vi "Dashboard Main.vi"() -> ()   [LabVIEW 2023]
uses:
  <vilib>/Rock Robotics/Network Tables/NT Read Numeric Array.vi
  <vilib>/Rock Robotics/Network Tables/NT Write Boolean.vi
  <vilib>/Rock Robotics/Network Tables/NT Write Number.vi
panel:
  out "Camera Perf":string
  in  "Camera Settings":T1={"Frame Rate"=30, "Compression"=30, "Size"=1, "DB Camera Config"=FALSE} {"Frame Rate" scale=1.0..30.0; "Compression" scale=100.0..-1.0; "Size" items=["640x480", "320x240", "160x120"]}
  in  "TCP":refnum<k5>
  out "Robot IP":string
  in  "Dashboard Tab":enum32{"Kilroy", "Variables", "Drive", "Basic"}(tab)
  in  "Auto Command Options":string(combo)
  in  "Demo Mode Enabled":bool
  in  "Auto Delay (seconds)":dbl(knob) min=0.0 max=5.0 scale=0.0..5.0 scale format="%#.2g"
  in  "Auto Selection":string(combo)
  in  "Auto Enabled":bool
  out "Tree":string(tree)
  in  "Select Auto":string(combo)="Select Autonomous ..."
  out "NT Connection":bool
  out "MotorChart R":cluster{"Numeric":dbl, "Numeric":dbl}(graph)
  out "MotorChart L":cluster{"Numeric":dbl, "Numeric":dbl}(graph)
  out "MotorSliders R":cluster{"MotorSlide1":dbl, "MotorSlide2":dbl} {"MotorSlide2" scale=-1.0..1.0 scale format="%#_2e"; "MotorSlide1" scale=-1.0..1.0 scale format="%#_2e"}
  out "MotorSliders L":cluster{"MotorSlide1":dbl, "MotorSlide2":dbl} {"MotorSlide2" scale=-1.0..1.0 scale format="%#_2e"; "MotorSlide1" scale=-1.0..1.0 scale format="%#_2e"}
  out "JS1 Z":dbl(slide) scale=-1.0..1.0 scale format="%#_2e"
  out "JS1 Graph":cluster{"X":dbl, "Y":dbl}[](graph)
  out "JS1 Buttons":T2
  out "JS2 Z":dbl(slide) scale=-1.0..1.0 scale format="%#_2e"
  out "JS2 Graph":cluster{"X":dbl, "Y":dbl}[](graph)
  out "JS2 Buttons":T2
  out "Mode":T3(ring)=enum."Auto Disabled"
  in  "DB/String 9":string
  in  "DB/String 8":string
  in  "DB/String 7":string
  in  "DB/String 6":string
  in  "DB/String 5":string
  in  "DB/String 4":string
  in  "DB/String 3":string
  in  "DB/String 2":string
  in  "DB/String 1":string
  in  "DB/String 0":string
  in  "DB/Slider 0":dbl(slide) scale=0.0..5.0
  in  "DB/Slider 1":dbl(slide) scale=0.0..5.0
  in  "DB/Slider 2":dbl(slide) scale=0.0..5.0
  in  "DB/Slider 3":dbl(slide) scale=0.0..5.0
  out "DB/LED 3":bool
  out "DB/LED 2":bool
  out "DB/LED 1":bool
  out "DB/LED 0":bool
  in  "DB/Button 3":bool
  in  "DB/Button 2":bool
  in  "DB/Button 1":bool
  in  "DB/Button 0":bool
  out "Camera Image":T4(plugin-control)
  out "Background":bool
  in  "Camera Name":string(combo)="No Camera Selection"
  # "HW"
  # "Joysticks"
  # "Drive Motors"
  # "Front"
  # "Right"
  # "Left"
  # "Back"
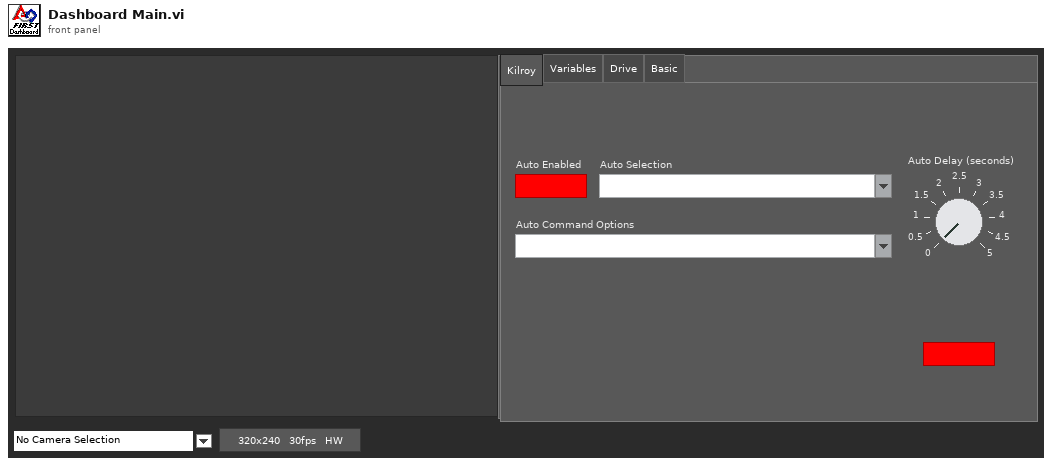
[diagram p1: front panel]
types:
  T1 = cluster{"Frame Rate":i32, "Compression":i32, "Size":u16, "DB Camera Config":bool}
  T2 = cluster{bool, bool, bool, bool, bool, bool, bool, bool, bool, bool, bool, bool}
  T3 = enum8{"Tele-Op Disabled", "Tele-Op Enabled", "Auto Disabled", "Auto Enabled", "Test Disabled", "Test Enabled", "Disconnected", "No Code", "E-Stop"}
  T4 = typedef "IMAQ Image.ctl" = refnum<image>
  T5 = cluster{"Save Path":path, "Interval (s)":dbl, "Keep":i32}
  T6 = typedef "Image Type" = u32
  T7 = cluster{"Camera Image":refnum<vi>, "Dashboard Tab":refnum<vi>, "Background":refnum<vi>, "Tree":refnum<vi>, "Camera Settings":refnum<vi>, "Camera Name":refnum<vi>, "Camera Perf":refnum<vi>}
  T8 = cluster{"Shift":bool, "Ctrl":bool, "Alt":bool, "Cmd":bool, "Opt":bool}
  T9 = cluster{"Error Strings":string, "Disable Counts":cluster{u16, u16}, "Rail Faults":cluster{u16, u16, u16}, "Robot IP":string, "DB Mode":u8, "Event Info":cluster{"Name":string, "Type":u8, "Number":u16, "Replay":u8}}
  T10 = cluster{"Storage":cluster{"Disk Free":u64, "RAM Block":u32, "RAM free":u32}, "CPU Utilization":cluster{"CPU % ISR":sgl, "CPU % Time Crit":sgl, "CPU % Timed Str":sgl, "CPU % High":sgl, "CPU % Above":sgl, "CPU % Normal":sgl, "CPU % Low":sgl}, "CAN":cluster{"% Bus Utilization":sgl, "Bus Off Cnt":u32, "TX_FIFO Full Cnt":u32, "Receive Error Cnt":u8, "Transmit Error Cnt":u8}, "HID":cluster{"HID Outputs":u32, "Rumble Low":u16, "Rumble High":u16}[]}
  T11 = cluster{"Status bits":cluster{"Test Mode":bool, "Autonomous":bool, "Enabled":bool, "Code Start":bool, "Brownout":bool, "Reserved 2":bool, "Reserved 3":bool, "E-Stop":bool}, "Code Trace":cluster{"Disabled":bool, "TeleOp":bool, "Auto":bool, "Test":bool}, "Controller Type":enum16{"unknown", "cRIO", "roboRio"}, "Code?":enum16{"unknown", "noCode", "code"}, "Battery V":dbl}
  T12 = cluster{"Control Bits":cluster{"TestMode":bool, "Autonomous":bool, "Enabled":bool, "FMS Present":bool, bool, bool, bool, "E-Stop":bool}, "Team Station ":u8, "Countdown":sgl, "Joystick Values":cluster{"Axes":dbl[], "Buttons":bool[], "POVs":i16[]}[]}
  T13 = cluster{"Axes":dbl[], "Buttons":bool[], "POVs":i16[]}[]
  T14 = cluster{"Axes":dbl[], "Buttons":bool[], "POVs":i16[]}
  T15 = cluster{"Buttons[0]":bool, "Buttons[1]":bool, "Buttons[2]":bool, "Buttons[3]":bool, "Buttons[4]":bool, "Buttons[5]":bool, "Buttons[6]":bool, "Buttons[7]":bool, "Buttons[8]":bool, "Buttons[9]":bool, "Buttons[10]":bool, "Buttons[11]":bool}
  T16 = cluster{"Camera Name":string, "Camera File Name":string, "Saved DB Images Info":cluster{"Save Path":path, "Interval (s)":dbl, "Keep":i32}}
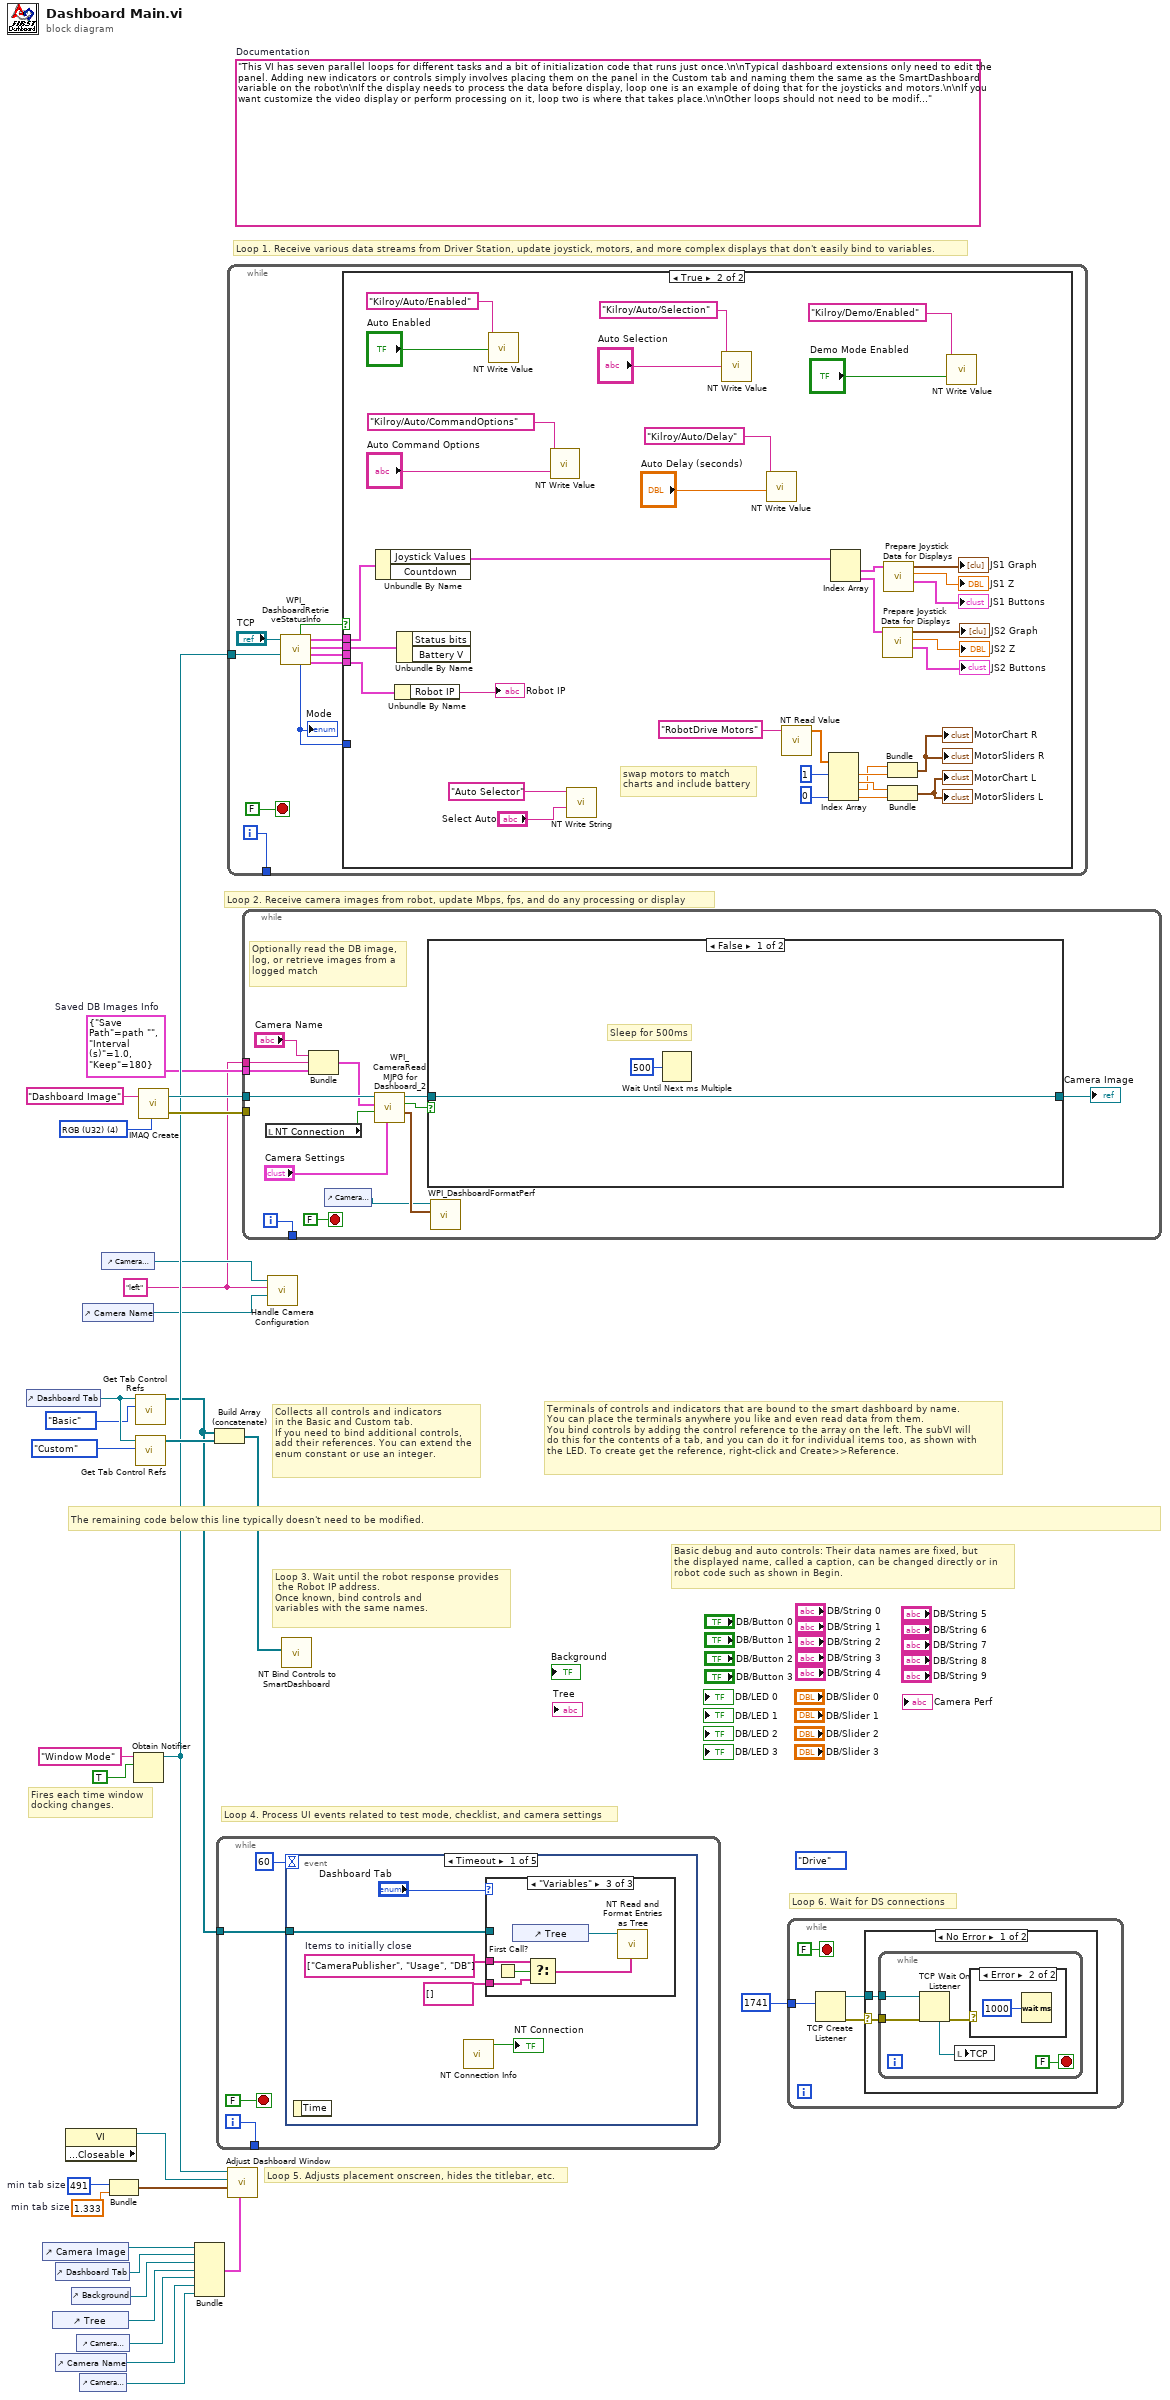
[diagram p0: block diagram]
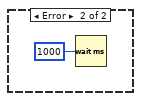
[diagram p3: hidden frame]
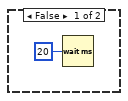
[diagram p4: hidden frame]
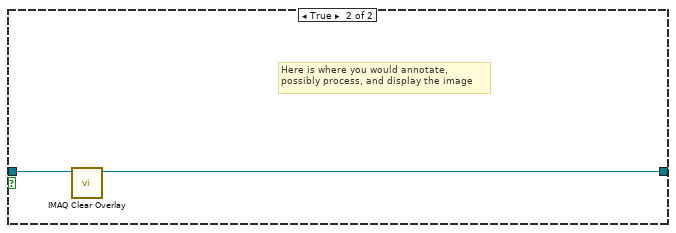
[diagram p5: hidden frame]
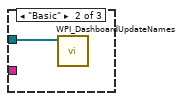
[diagram p7: hidden frame]
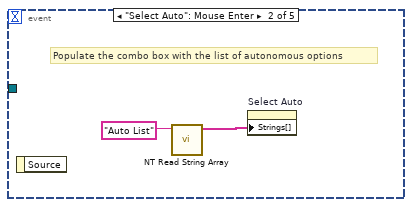
[diagram p8: hidden frame]
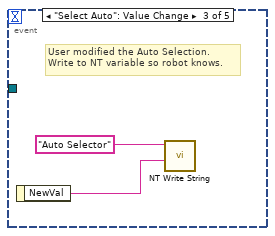
[diagram p9: hidden frame]
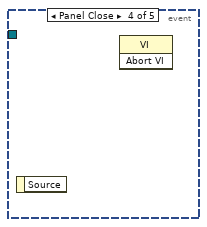
[diagram p10: hidden frame]
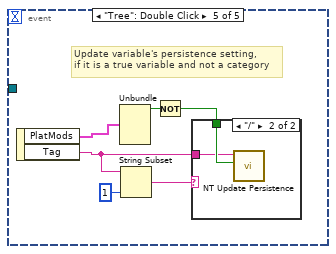
[diagram p11: hidden frame]
diagram:
  w2 = "left" ("Camera File Name")
  w3 = T5 {"Save Path"=path "", "Interval (s)"=1.0, "Keep"=180}  # Saved DB Images Info
  (unwired) enum32{"Drive", "Basic", "Custom", "Variables"}."Drive" ("Dashboard Tab")
  w18 = 491  # min tab size
  w17 = 1.333  # min tab size
  (unwired) "This VI has seven parallel loops for different tasks and a bit of initialization code that runs just once.\n\nTypical dashboard extensions only need to edit the panel. Adding new indicators or controls simply involves placing them on the panel in the Custom tab and naming them the same as the SmartDashboard variable on the robot\n\nIf the display needs to process the data before display, loop one is an example of doing that for the joysticks and motors.\n\nIf you want customize the video display or perform processing on it, loop two is where that takes place.\n\nOther loops should not need to be modified. They are pretty standard, and document the task they perform."  # Documentation
  w30 = T6 4 items=["Grayscale (U8)", "Grayscale (I16)", "Grayscale (SGL)", "Complex (CSG)", "RGB (U32)", "HSL (U32)", "RGB (U64)"] ("Image Type")
  # "Loop 6. Wait for DS connections"
  # "Basic debug and auto controls: Their data names are fixed, but\nthe displayed name, called a caption, can be changed directly or in\nrobot code such as shown in Begin."
  # "Fires each time window\ndocking changes."
  # "Collects all controls and indicators\nin the Basic and Custom tab.\nIf you need to bind additional controls,\nadd their references. You can extend the\nenum constant or use an integer."
  # "The remaining code below this line typically doesn't need to be modified."
  # "Loop 4. Process UI events related to test mode, checklist, and camera settings"
  # "Terminals of controls and indicators that are bound to the smart dashboard by name.\nYou can place the terminals anywhere you like and even read data from them.\nYou bind controls by adding the control reference to the array on the left. The subVI will\ndo this for the contents of a tab, and you can do it for individual items too, as shown with\nthe LED. To create get the reference, right-click and Create>>Reference."
  # "Loop 3. Wait until the robot response provides\n the Robot IP address.\nOnce known, bind controls and\nvariables with the same names."
  # "Loop 5. Adjusts placement onscreen, hides the titlebar, etc."
  # "Loop 1. Receive various data streams from Driver Station, update joystick, motors, and more complex displays that don't easily bind to variables."
  # "Loop 2. Receive camera images from robot, update Mbps, fps, and do any processing or display"
  n1 = control-ref of="Dashboard Tab"() -> (w23:refnum<vi>)
  n2 = control-ref of="Camera Image"() -> (w20:refnum<vi>)
  n3 = control-ref of="Tree"() -> (w9:refnum<vi>)
  n4 = control-ref of="Dashboard Tab"() -> (w19:refnum<vi>)
  n5 = control-ref of="Camera Name"() -> (w7:refnum<vi>)
  n6 = property class="VI" props=["Front Panel.Closeable"]() -> (reference out=w24:refnum<vi>)  [unwired: 2 in, 2 out]
  n7 = control-ref of="Background"() -> (w15:refnum<vi>)
  n8 = control-ref of="Camera Settings"() -> (w8:refnum<vi>)
  n9 = control-ref of="Camera Perf"() -> (w6:refnum<vi>)
  n10 = control-ref of="Camera Name"() -> (w11:refnum<vi>)
  n11 = control-ref of="Camera Settings"() -> (w12:refnum<vi>)
  n12 = Bundle("min tab size"=w18, "min tab size"=w17) -> (w16:cluster{"min tab size":i32, "min tab size":dbl})  [unwired: 1 in]
  n13 = Obtain Notifier(name (unnamed)="Window Mode", notification data type=TRUE) -> (notifier out=w13:refnum<notifier>)  [unwired: 2 in, 2 out]
  n14 = call <vilib>:"Get Tab Control Refs.vi"("Page Index"=enum32{"Drive", "Basic", "Custom", "Variables"}."Basic" ("Dashboard Tab"), "TabControl in"=w23) -> ("ControlsOnPage"=w10:refnum<vi>[])  [unwired: 9 in]
  n15 = call <vilib>:"Get Tab Control Refs.vi"("Page Index"=enum32{"Drive", "Basic", "Custom", "Variables"}."Custom" ("Dashboard Tab"), "TabControl in"=w23) -> ("ControlsOnPage"=w22:refnum<vi>[])  [unwired: 9 in]
  n16 = call "IMAQ Create"("Image Name"="Dashboard Image", "Image Type"=w30) -> ("New Image"=w28:T4, "error out"=w27:errorcluster)  [unwired: 2 in, 1 out]
  n17 = Bundle("Camera Image"=w20, "Dashboard Tab"=w19, "Background"=w15, "Tree"=w9, "Camera Settings"=w8, "Camera Name"=w7, "Camera Perf"=w6) -> (w14:T7)  [unwired: 1 in]
  n18 = Build Array (concatenate)(w10, w22) -> (w21:refnum<vi>[])
  n19 = while {
    tunnel: [w32] -> _
    tunnel: w10 -> [w31]
    i -> [w32]
    stop <- FALSE stop-if-true
    n20 = event shown="[0] Timeout" {
      selector: _ -> [_ _ _ _ _]
      dyn-events: _ -> [_ _ _ _ _]
      timeout: u32 60 ("milliseconds to wait") -> [_ _ _ _ _]
      tunnel: w31 -> [w38 _ _ _ _]
      event Timeout {
        w37 = string[] ["CameraPublisher", "Usage", "DB"]  # Items to initially close
        n21 = event-data() -> ()  [unwired: 1 in, 1 out]
        n22 = call <vilib>:"NT Connection Info.vi"() -> ("Connected"=→"NT Connection":bool)  [unwired: 11 in]
        n23 = case shown="\"Variables\"" "Dashboard Tab" {
          tunnel: w38 -> [_ w40 _]
          tunnel: w37 -> [_ _ w43]
          tunnel: string[] [] -> [_ _ w42]
          frame "Kilroy", Default {
          }
          frame "Basic" {
            n24 = call <vilib>:"WPI_DashboardUpdateNames.vi"("Controls on Tab"=w40) -> ()  [unwired: 11 in]
          }
          frame "Variables" {
            n25 = First Call?() -> (First Call?: T/F=w44:bool)
            n26 = control-ref of="Tree"() -> (w45:refnum<vi>)
            n27 = Select(t=w43, s=w44, f=w42) -> (s? t:f=w41:string[])
            n28 = call <vilib>:"NT Read and Format Entries as Tree.vi"("Tags to  Close"=w41, "Tree Refnum"=w45) -> ()  [unwired: 8 in, 2 out]
          }
        }
      }
      event "Select Auto": Mouse Enter {
        # "Populate the combo box with the list of autonomous options"
        n29 = event-data() -> ()  [unwired: 1 in, 1 out]
        n30 = call <vilib>:"NT Read String Array.vi"("name"="Auto List" ("Name")) -> ("value"=w46:string[])  [unwired: 8 in, 2 out]
        n31 = property on="Select Auto" class="CmbBox"("Strings[]"=w46) -> ()  [unwired: 2 in, 2 out]
      }
      event "Select Auto": Value Change {
        # "User modified the Auto Selection.\nWrite to NT variable so robot knows."
        n32 = event-data() -> ("NewVal"=w48:string)  [unwired: 1 in]
        n33 = call <vilib>:"NT Write String.vi"("value"=w48, "name"="Auto Selector" ("Name")) -> ()  [unwired: 9 in, 1 out]
      }
      event Panel Close {
        n34 = event-data() -> ()  [unwired: 1 in, 1 out]
        n35 = invoke class="VI" method="Abort VI"() -> ()  [unwired: 3 in, 3 out]
      }
      event "Tree": Double Click {
        # "Update variable's persistence setting,\nif it is a true variable and not a category"
        n36 = event-data() -> ("PlatMods"=w51:T8, "Tag"=w50:string)  [unwired: 1 in]
        n37 = Unbundle(w51) -> ("Shift"=w55:bool)  [unwired: 4 out]
        n38 = String Subset(string=w50, length (rest)=1 ("length (rest)")) -> (substring=w52:string)  [unwired: 1 in]
        n39 = Not(x=w55) -> (.not. x?=w54:bool)
        n40 = case shown="\"/\"" w52 {
          tunnel: w54 -> [_ w57]
          tunnel: w50 -> [_ w56]
          frame Default {
          }
          frame "/" {
            n41 = call <vilib>:"NT Update Persistence.vi"("Persistence"=w57, "Name"=w56) -> ()  [unwired: 9 in, 1 out]
          }
        }
      }
    }
  }
  n42 = while {
    tunnel: [w66] -> _
    tunnel: w13 -> [w58]
    i -> [w66]
    stop <- FALSE stop-if-true
    n43 = call <vilib>:"WPI_DashboardRetrieveStatusInfo.vi"("Window Mode Notifier"=w58, "TCP Cnx"="TCP") -> ("Power and Errors"=w61:T9, "Robot Metrics"=w64:T10, "Status Info"=w65:T11, "Control Info"=w62:T12, "Robot Mode"=w60:T3, "Process?"=w63:bool)  [unwired: 4 in]
    "Mode" <- w60
    n44 = case shown="True" w63 {
      tunnel: w65 -> [_ w103]
      tunnel: w64 -> [_ _]
      tunnel: w62 -> [_ w102]
      tunnel: w61 -> [_ w101]
      tunnel: w60 -> [_ _]
      frame False {
        n45 = Wait (ms)(milliseconds to wait=u32 20) -> ()  [unwired: 1 out]
      }
      frame True {
        # "swap motors to match\ncharts and include battery"
        n46 = Unbundle By Name(w102) -> ("Joystick Values"=w92:T13)  [unwired: 1 out]
        n47 = Unbundle By Name(w101) -> ("Robot IP"=→"Robot IP":string)
        n48 = Unbundle By Name(w103) -> ()  [unwired: 2 out]
        n49 = call-poly <vilib>:"NT Write Value.vi"("value"="Auto Enabled", "name"="Kilroy/Auto/Enabled") -> ()  [unwired: 9 in, 1 out]
        n50 = call-poly <vilib>:"NT Write Value.vi"("value"="Auto Command Options", "name"="Kilroy/Auto/CommandOptions") -> ()  [unwired: 9 in, 1 out]
        n51 = call <vilib>:"NT Write String.vi"("value"="Select Auto", "name"="Auto Selector" ("Name")) -> ()  [unwired: 9 in, 1 out]
        n52 = call-poly <vilib>:"NT Write Value.vi"("value"="Auto Selection", "name"="Kilroy/Auto/Selection") -> ()  [unwired: 9 in, 1 out]
        n53 = call-poly <vilib>:"NT Write Value.vi"("value"="Auto Delay (seconds)", "name"="Kilroy/Auto/Delay") -> ()  [unwired: 9 in, 1 out]
        n54 = call-poly <vilib>:"NT Read Value.vi"("name"="RobotDrive Motors" ("Name")) -> ("value"=w82:dbl[])  [unwired: 8 in, 2 out]
        n55 = Index Array(array=w82, index #1=1, index #4=0) -> (element #1=w96:dbl, element #2=w97:dbl, element #3=w95:dbl, element #4=w100:dbl)  [unwired: 2 in]
        n56 = Index Array(array=w92) -> (element #1=w91:T14, element #2=w87:T14)  [unwired: 2 in]
        n57 = call "Prepare Joystick Data for Displays.vi"("Joystick Values"=w87) -> ("Buttons"=→"JS2 Buttons":T15, "Z Axis"=→"JS2 Z":dbl, "Cartesian Data"=→"JS2 Graph":cluster{"X axis":dbl, "X axis":dbl}[])  [unwired: 8 in]
        n58 = call "Prepare Joystick Data for Displays.vi"("Joystick Values"=w91) -> ("Buttons"=→"JS1 Buttons":T15, "Z Axis"=→"JS1 Z":dbl, "Cartesian Data"=→"JS1 Graph":cluster{"X axis":dbl, "X axis":dbl}[])  [unwired: 8 in]
        n59 = Bundle("Numeric"=w95, "Numeric"=w96) -> (→"MotorChart R" →"MotorSliders R":cluster{"Numeric":dbl, "Numeric":dbl})  [unwired: 1 in]
        n60 = Bundle("Numeric"=w97, "Numeric"=w100) -> (→"MotorChart L" →"MotorSliders L":cluster{"Numeric":dbl, "Numeric":dbl})  [unwired: 1 in]
        n61 = call-poly <vilib>:"NT Write Value.vi"("value"="Demo Mode Enabled", "name"="Kilroy/Demo/Enabled") -> ()  [unwired: 9 in, 1 out]
      }
    }
  }
  n62 = call "Adjust Dashboard Window.vi"("Sizing Refnums"=w14, "Size Constraints"=w16, "VI"=w24, "WIn Mode"=w13) -> ()  [unwired: 8 in]
  n63 = while {
    tunnel: w28 -> [w115]
    tunnel: w27 -> [_]
    tunnel: [w116] -> _
    tunnel: w3 -> [w109]
    tunnel: w2 -> [w106]
    i -> [w116]
    stop <- FALSE stop-if-true
    # "Optionally read the DB image,\nlog, or retrieve images from a\nlogged match"
    n64 = local read "NT Connection"() -> (w110:bool)
    n65 = Bundle("Camera Name"="Camera Name", "Camera File Name"=w106, "Saved DB Images Info"=w109) -> (w108:T16)  [unwired: 1 in]
    n66 = control-ref of="Camera Perf"() -> (w104:refnum<vi>)
    n67 = call <vilib>:"WPI_CameraRead MJPG for Dashboard_2.vi"("Camera Settings"="Camera Settings", "NT Connection"=w110, "Capture Info"=w108, "Image in"=w115) -> ("perf info"=w105:cluster{"Bandwidth (Mbps)":dbl, "fps":dbl}, "Active"=w113:bool, "Image\\ out"=w114:T4)  [unwired: 5 in]
    n68 = case shown="False" w113 {
      tunnel: w114 -> [w118 w121]
      tunnel: [w118 w120] -> w111
      frame False {
        # "Sleep for 500ms"
        n69 = Wait Until Next ms Multiple(millisecond multiple=u32 500) -> ()  [unwired: 1 out]
      }
      frame True {
        # "Here is where you would annotate,\npossibly process, and display the image"
        n70 = call "IMAQ Clear Overlay"("Image"=w121) -> ("Image Out"=w120:T4)  [unwired: 2 in, 8 out]
      }
    }
    "Camera Image" <- w111
    n71 = call <vilib>:"WPI_DashboardFormatPerf.vi"("Performance"=w105, "String in"=w104) -> ()  [unwired: 10 in]
  }
  n72 = call "Handle Camera Configuration.vi"("CameraNameRef"=w11, "Display Name"=w2, "ClusterRef"=w12) -> ()  [unwired: 9 in]
  n73 = call <vilib>:"NT Bind Controls to SmartDashboard.vi"("Bound Control Refs"=w21) -> ()  [unwired: 11 in]
  n74 = while {
    tunnel: u16 1741 ("timeout ms (25000)") -> [w123]
    stop <- FALSE stop-if-true
    n75 = TCP Create Listener(10:w123) -> (0:w122:errorcluster, 3:w124:refnum<k5>)  [unwired: 4 in, 1 out]
    n76 = case shown="No Error" w122 {
      selector: w122 -> [w126 _]
      tunnel: w124 -> [w127 _]
      frame No Error {
        n77 = while {
          tunnel: w127 -> [w130]
          tunnel: w126 -> [w129]
          stop <- FALSE stop-if-true
          n78 = TCP Wait On Listener(8:w129, 11:w130) -> (0:w131:errorcluster, 4:w132:refnum<k5>)  [unwired: 2 in, 3 out]
          n79 = local write "TCP"(w132) -> ()
          n80 = case shown="Error" w131 {
            frame No Error {
            }
            frame Error {
              n81 = Wait (ms)(milliseconds to wait=u32 1000) -> ()  [unwired: 1 out]
            }
          }
        }
      }
      frame Error {
        n82 = Wait (ms)(milliseconds to wait=u32 1000) -> ()  [unwired: 1 out]
      }
    }
  }
